vi "rcpacini_e_resize_diagram.vi"(6 "Variant in":variant, 7 "Shift Pressed?":bool, 8 "error in (no error)":errorcluster, 10 "QD Combo Box Ref":refnum<vi>, 11 "QD Launch VI Ref":refnum<vi>) -> (0 "error out":errorcluster, 4 "Variant out":variant)   [LabVIEW 2019]
doc: "Resizes the block diagram window to content. (Front panel focus does nothing).\n\nCreated by: Ryan Pacini\n\nDefault Shortcut - [E]"
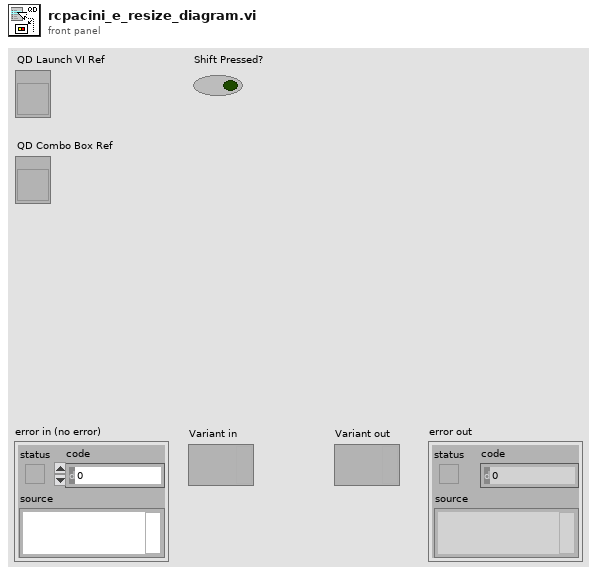
[diagram p1: front panel]
types:
  T1 = typedef "LVRectTypeDef.ctl" = cluster{"Left":i16, "Top":i16, "Right":i16, "Bottom":i16}
  T2 = typedef "LVAllMonitorsDisplayTypeDef.ctl" = cluster{"Bounds":cluster{"Left":i16, "Top":i16, "Right":i16, "Bottom":i16}, "Depth":i16}[]
  T3 = typedef "LVBoundsTypeDef.ctl" = cluster{"Width":u32, "Height":u32}
  T4 = cluster{"Left":i16, "Top":i16, "Right":i16, "Bottom":i16}
  T5 = typedef "LVPointTypeDef.ctl" = cluster{"Horizontal":i16, "Vertical":i16}
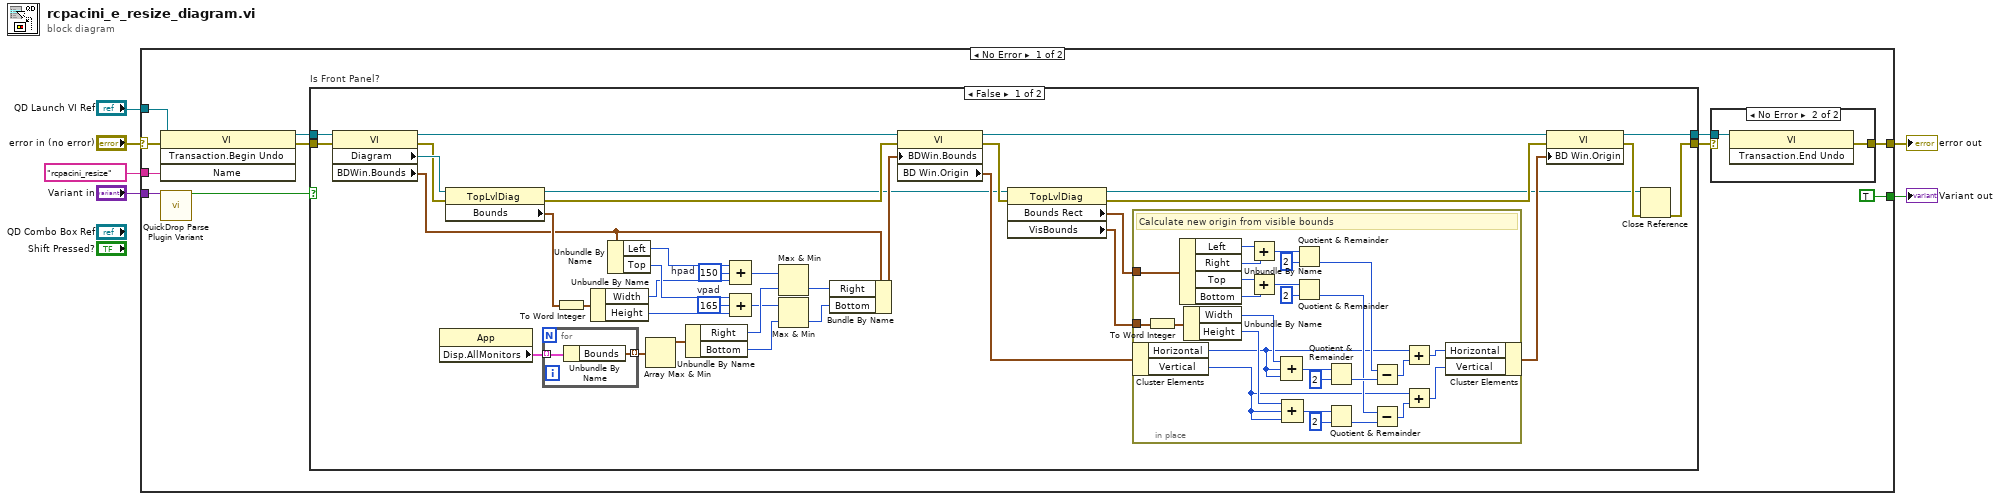
[diagram p0: block diagram]
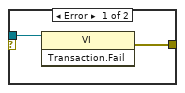
[diagram p3: hidden frame]
diagram:
  n1 = case shown="No Error" "error in (no error)" {
    selector: "error in (no error)" -> [w17 w89]
    tunnel: [w16 w89] -> w1
    tunnel: "QD Launch VI Ref" -> [w11 _]
    tunnel: "rcpacini_resize" ("Undo Name") -> [w15 _]
    tunnel: "Variant in" -> [w13 _]
    tunnel: [TRUE _] -> w2
    frame No Error {
      n2 = invoke class="VI" method="Transaction.Begin Undo"(reference=w11, error in=w17, "Name"=w15) -> (reference out=w9:refnum<vi>, error out=w10:errorcluster)  [unwired: 1 in, 2 out]
      n3 = call <vilib>:"QuickDrop Parse Plugin Variant.vi"("QDKS Variant in"=w13) -> ("QD Launch VI Panel?"=w7:bool)  [unwired: 12 in, 2 out]
      n4 = case "Is Front Panel?" shown="False" w7 {
        tunnel: [w21 w84] -> w12
        tunnel: w10 -> [w20 w84]
        tunnel: w9 -> [w19 w83]
        tunnel: [w18 w83] -> w8
        frame False {
          w34 = i16 165  # vpad
          w44 = i16 150  # hpad
          n5 = property on="Property Node" class="VI"(reference=w19, error in=w20) -> (error out=w40:errorcluster, "Diagram"=w49:refnum<vi>, "BDWin.Bounds"=w25:T1)  [unwired: 1 out]
          n6 = property class="App"() -> ("Disp.AllMonitors"=w53:T2)  [unwired: 2 in, 2 out]
          n7 = property on="Property Node" class="TopLvlDiag"(reference=w49, error in=w40) -> (reference out=w23:refnum<vi>, error out=w41:errorcluster, "Bounds"=w42:T3)
          n8 = for {
            tunnel: w53 -> [w82] mode=indexing
            tunnel: [w81] -> w52 mode=indexing
            n9 = Unbundle By Name(w82) -> ("Bounds"=w81:T4)
          }
          n10 = To Word Integer(number=w42) -> (16bit integer=w31:cluster{"Width":i16, "Height":i16})
          n11 = Unbundle By Name(w31) -> ("Width"=w29:i16, "Height"=w30:i16)
          n12 = Unbundle By Name(w25) -> ("Left"=w32:i16, "Top"=w33:i16)
          n13 = Array Max & Min(array=w52) -> (max value=w35:T4)  [unwired: 3 out]
          n14 = Unbundle By Name(w35) -> ("Right"=w51:i16, "Bottom"=w50:i16)
          n15 = Compound Arithmetic op=ADD(w32, w44, w29) -> (w39:i16)
          n16 = Compound Arithmetic op=ADD(w33, w34, w30) -> (w38:i16)
          n17 = Max & Min(x=w39, y=w51) -> (min(x,y)=w37:i16)  [unwired: 1 out]
          n18 = Max & Min(x=w38, y=w50) -> (min(x,y)=w36:i16)  [unwired: 1 out]
          n19 = Bundle By Name(cluster=w25, "Right"=w37, "Bottom"=w36) -> (w43:T1)
          n20 = property on="Property Node" class="VI"(reference=w19, error in=w41, "BDWin.Bounds"=w43) -> (reference out=w24:refnum<vi>, error out=w45:errorcluster, "BD Win.Origin"=w27:T5)
          n21 = property on="Property Node" class="TopLvlDiag"(reference=w23, error in=w45) -> (reference out=w22:refnum<vi>, error out=w47:errorcluster, "Bounds Rect"=w46:T1, "VisBounds"=w28:T3)
          n22 = in-place {
            in-place-border: w46 -> [w76]
            in-place-border: w28 -> [w64]
            # "Calculate new origin from visible bounds"
            n23 = in-place-cluster #1(w27) -> ("Horizontal"=w58:i16, "Vertical"=w57:i16)
            n24 = To Word Integer(number=w64) -> (16bit integer=w63:cluster{"Width":i16, "Height":i16})
            n25 = Unbundle By Name(w76) -> ("Left"=w80:i16, "Right"=w79:i16, "Top"=w78:i16, "Bottom"=w77:i16)
            n26 = Unbundle By Name(w63) -> ("Width"=w60:i16, "Height"=w62:i16)
            n27 = Add(x=w80, y=w79) -> (x+y=w75:i16)
            n28 = Add(x=w78, y=w77) -> (x+y=w74:i16)
            n29 = Compound Arithmetic op=ADD(w60, w58, w58) -> (w59:i16)
            n30 = Compound Arithmetic op=ADD(w62, w57, w57) -> (w61:i16)
            n31 = Quotient & Remainder(x=w75, y=i16 2) -> (floor(x/y)=w70:i16)  [unwired: 1 out]
            n32 = Quotient & Remainder(x=w74, y=i16 2) -> (floor(x/y)=w67:i16)  [unwired: 1 out]
            n33 = Quotient & Remainder(x=w59, y=i16 2) -> (floor(x/y)=w71:i16)  [unwired: 1 out]
            n34 = Quotient & Remainder(x=w61, y=i16 2) -> (floor(x/y)=w69:i16)  [unwired: 1 out]
            n35 = Subtract(x=w70, y=w71) -> (x-y=w66:i16)
            n36 = Subtract(x=w67, y=w69) -> (x-y=w65:i16)
            n37 = Add(x=w58, y=w66) -> (x+y=w56:i16)
            n38 = Add(x=w57, y=w65) -> (x+y=w55:i16)
            n39 = in-place-cluster #1("Horizontal"=w56, "Vertical"=w55) -> (w26:T5)
          }
          n40 = property on="Property Node" class="VI"(reference=w24, error in=w47, "BD Win.Origin"=w26) -> (reference out=w18:refnum<vi>, error out=w48:errorcluster)
          n41 = Close Reference(reference=w22, error in (no error)=w48) -> (error out=w21:errorcluster)
        }
        frame True {
        }
      }
      n42 = case shown="No Error" w12 {
        tunnel: w8 -> [w85 w87]
        tunnel: [w86 w88] -> w16
        frame Error {
          n43 = invoke class="VI" method="Transaction.Fail"(reference=w85) -> (error out=w86:errorcluster)  [unwired: 2 in, 2 out]
        }
        frame No Error {
          n44 = invoke class="VI" method="Transaction.End Undo"(reference=w87) -> (error out=w88:errorcluster)  [unwired: 2 in, 2 out]
        }
      }
    }
    frame Error {
    }
  }
  "error out" <- w1
  "Variant out" <- w2
